vi "telemetria3.vi"(11 "Output Array":string[][](array[string])) -> (0 "v3":dbl format="%.2f", 1 "sr v2":dbl format="%0.2f", 2 "v2":dbl format="%.2f", 3 "œr v1":dbl format="%0.2f", 4 "sr v3":dbl format="%0.2f", 5 "v 1":dbl format="%.2f", 6 "output cluster":T1, 7 "srednie sr":cluster{dbl, dbl}, 8 "raw":cluster{u16, u16, u16, u16, u16, u16})   [LabVIEW 2015]
uses:
  <vilib>/ptbypt/NI_PtbyPt.lvlib
panel:
  out "Result":string
  out "match + rest of string":string
  out "substring before match":string
  out "concatenated string":string
  out "element 3":string
  out "œr v1  2":dbl format="%0.2f"
  out "sr v2 2":dbl format="%0.2f"
  out "v 2":dbl format="%.2f"
  out "v2 2":dbl format="%.2f"
  out "sr v3 2":dbl format="%0.2f"
  out "v3  2":dbl format="%.2f"
  out "element 2":string
  out "element":string
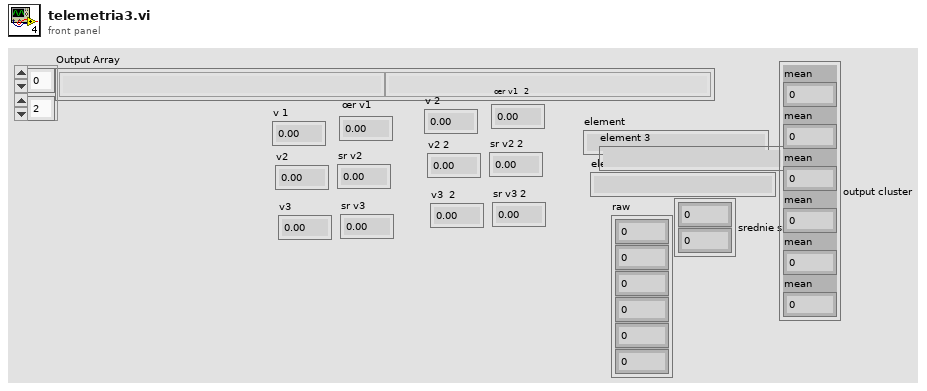
[diagram p1: front panel]
types:
  T1 = cluster{"mean":dbl, "mean":dbl, "mean":dbl, "mean":dbl, "mean":dbl, "mean":dbl}
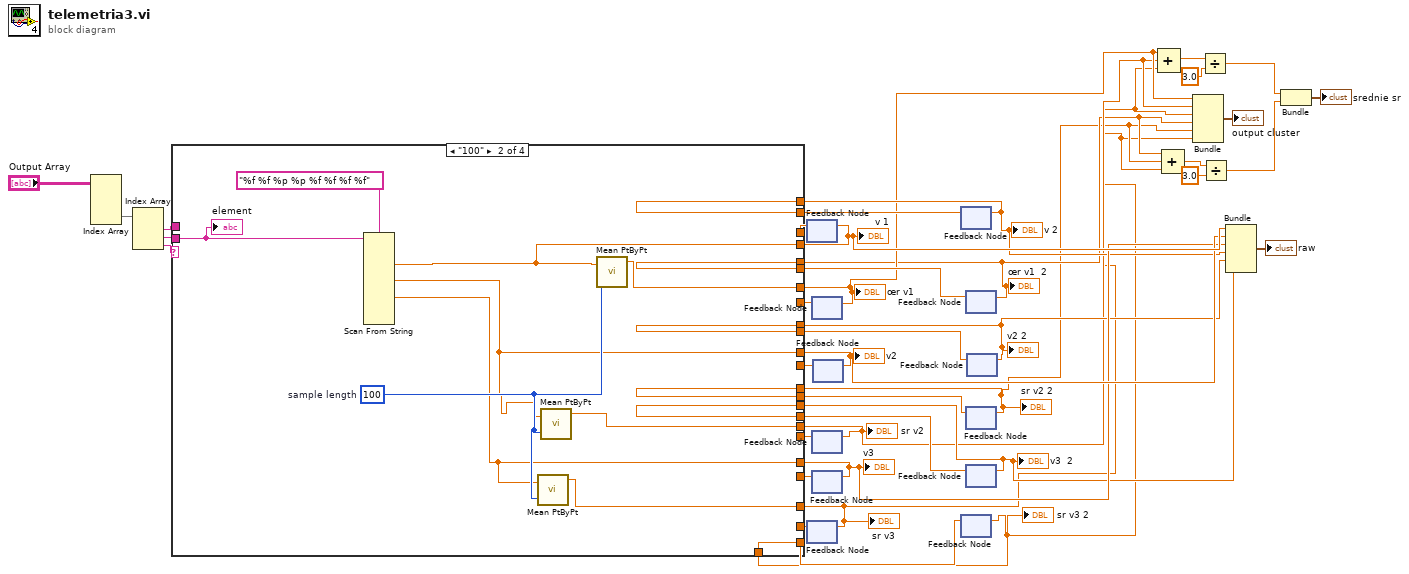
[diagram p0: block diagram]
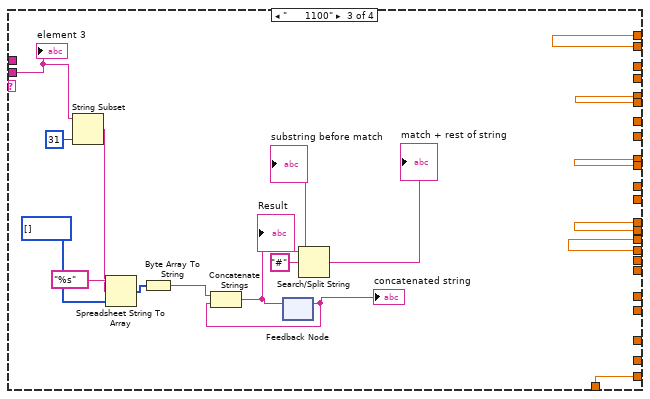
[diagram p3: hidden frame]
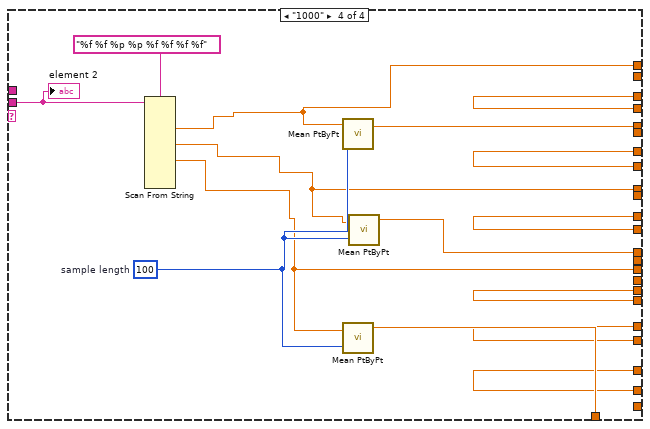
[diagram p4: hidden frame]
diagram:
  n1 = Index Array(array="Output Array") -> (element #2=w37:string[])  [unwired: 4 in, 1 out]
  n2 = Index Array(array=w37) -> (element #1=w30:string, element #2=w36:string, element #3=w35:string)  [unwired: 3 in]
  n3 = feedback #1() -> (w32:dbl)  [unwired: 1 in]
  n4 = feedback #2() -> (w28:dbl)  [unwired: 1 in]
  n5 = feedback #3() -> (w33:dbl)  [unwired: 1 in]
  n6 = feedback #4() -> (w34:dbl)  [unwired: 1 in]
  n7 = feedback #5() -> (w29:dbl)  [unwired: 1 in]
  n8 = feedback #6() -> (w31:dbl)  [unwired: 1 in]
  n9 = feedback #7() -> (w27:dbl)  [unwired: 1 in]
  n10 = feedback #8() -> (w22:dbl)  [unwired: 1 in]
  n11 = feedback #9() -> (w26:dbl)  [unwired: 1 in]
  n12 = feedback #10() -> (w24:dbl)  [unwired: 1 in]
  n13 = feedback #11() -> (w23:dbl)  [unwired: 1 in]
  n14 = feedback #12() -> (w25:dbl)  [unwired: 1 in]
  n15 = case shown="\"100\"" w35 {
    tunnel: w36 -> [_ w64 w75 w97]
    tunnel: [w49 w63 _ w93] -> w7
    tunnel: [w50 w62 _ w91] -> w6
    tunnel: w34 -> [w50 _ _ w91]
    tunnel: w33 -> [w49 _ _ w93]
    tunnel: [w48 w53 _ w94] -> w21
    tunnel: [w47 w52 _ w92] -> w20
    tunnel: w32 -> [w48 _ _ w94]
    tunnel: w31 -> [w47 _ _ w92]
    tunnel: w30 -> [_ _ _ _]
    tunnel: [w46 w51 _ w90] -> w19
    tunnel: [w45 w61 _ w89] -> w5
    tunnel: w29 -> [w46 _ _ w90]
    tunnel: w28 -> [w45 _ _ w89]
    tunnel: [w44 w60 w83 w86] -> w18
    tunnel: [w43 w59 w82 w87] -> w4
    tunnel: [w42 w58 w81 w85] -> w17
    tunnel: [w41 w57 w80 w96] -> w3
    tunnel: [w40 w56 w79 w84] -> w16
    tunnel: [w39 w55 w78 w95] -> w2
    tunnel: w27 -> [w44 w60 w83 _]
    tunnel: w26 -> [w43 w59 w82 _]
    tunnel: w25 -> [w42 w58 w81 _]
    tunnel: w24 -> [w41 w57 w80 _]
    tunnel: w23 -> [w40 w56 w79 _]
    tunnel: w22 -> [w39 w55 w78 _]
    frame "False", Default {
    }
    frame "100" {
      w54 = 100  # sample length
      n16 = Scan From String(format string="%f %f %p %p %f %f %f %f", input string=w64) -> (output 1=w53:dbl, output 3=w52:dbl, output 5=w51:dbl)  [unwired: 15 in, 3 out]
      n17 = call <vilib>:"Mean PtByPt.vi"("x"=w51, "sample length"=w54) -> ("mean"=w61:dbl)  [unwired: 2 in, 1 out]
      n18 = call <vilib>:"Mean PtByPt.vi"("x"=w52, "sample length"=w54) -> ("mean"=w62:dbl)  [unwired: 2 in, 1 out]
      n19 = call <vilib>:"Mean PtByPt.vi"("x"=w53, "sample length"=w54) -> ("mean"=w63:dbl)  [unwired: 2 in, 1 out]
      "element" <- w64
    }
    frame "      1100" {
      n20 = String Subset(string=w75, length (rest)=31 ("length (rest)")) -> (substring=w73:string)  [unwired: 1 in]
      n21 = Spreadsheet String To Array(format string="%s", spreadsheet string=w73, array type (2D Dbl)=u8[] [] ("unsigned byte array")) -> (array=w72:u8[])  [unwired: 1 in]
      n22 = Byte Array To String(unsigned byte array=w72) -> (string=w66:string)
      n23 = feedback #13() -> (w71:string)  [unwired: 1 in]
      "concatenated string" <- w71
      n24 = Concatenate Strings(w66, w71) -> (w70:string)
      n25 = feedback-in #13(w70) -> ()
      n26 = Search/Split String(string=w70, search string/char (-)="#") -> (substring before match=→"substring before match":string, match + rest of string=→"match + rest of string":string)  [unwired: 1 in, 1 out]
      "element 3" <- w75
    }
    frame "1000" {
      w88 = 100  # sample length
      n27 = Scan From String(format string="%f %f %p %p %f %f %f %f", input string=w97) -> (output 1=w86:dbl, output 3=w85:dbl, output 5=w84:dbl)  [unwired: 15 in, 3 out]
      n28 = call <vilib>:"Mean PtByPt.vi"("x"=w86, "sample length"=w88) -> ("mean"=w87:dbl)  [unwired: 2 in, 1 out]
      n29 = call <vilib>:"Mean PtByPt.vi"("x"=w84, "sample length"=w88) -> ("mean"=w95:dbl)  [unwired: 2 in, 1 out]
      n30 = call <vilib>:"Mean PtByPt.vi"("x"=w85, "sample length"=w88) -> ("mean"=w96:dbl)  [unwired: 2 in, 1 out]
      "element 2" <- w97
    }
  }
  "œr v1" <- w7
  "sr v2" <- w6
  "v 1" <- w21
  "v2" <- w20
  "sr v3" <- w5
  "v3" <- w19
  "œr v1  2" <- w4
  "sr v2 2" <- w3
  "v 2" <- w18
  "v2 2" <- w17
  "sr v3 2" <- w2
  "v3  2" <- w16
  n31 = feedback-in #1(w21) -> ()
  n32 = feedback-in #2(w5) -> ()
  n33 = feedback-in #3(w7) -> ()
  n34 = feedback-in #4(w6) -> ()
  n35 = feedback-in #5(w19) -> ()
  n36 = feedback-in #6(w20) -> ()
  n37 = feedback-in #7(w18) -> ()
  n38 = feedback-in #8(w2) -> ()
  n39 = feedback-in #9(w4) -> ()
  n40 = feedback-in #10(w3) -> ()
  n41 = feedback-in #11(w16) -> ()
  n42 = feedback-in #12(w17) -> ()
  n43 = Compound Arithmetic op=ADD(w7, w6, w5) -> (w14:dbl)
  n44 = Compound Arithmetic op=ADD(w4, w3, w2) -> (w13:dbl)
  n45 = Bundle("mean"=w7, "mean"=w6, "mean"=w5, "mean"=w4, "mean"=w3, "mean"=w2) -> (→"output cluster":T1)  [unwired: 1 in]
  n46 = Divide(x=w14, y=3.0) -> (x/y=w10:dbl)
  n47 = Divide(x=w13, y=3.0) -> (x/y=w9:dbl)
  n48 = Bundle(w21, w20, w19, w18, w17, w16) -> (→"raw":cluster{dbl, dbl, dbl, dbl, dbl, dbl})  [unwired: 1 in]
  n49 = Bundle(w10, w9) -> (→"srednie sr":cluster{dbl, dbl})  [unwired: 1 in]
